vi "DL-Initialize Logging.vi"(0 "Configuration":cluster{"Stop":bool, "Config":T1}, 11 "error in (no error)":errorcluster) -> (3 "RPcoX":refnum<k7>, 4 "task":refnum<k21>, 8 "Npts":i32, 13 "Config.T (s)":dbl, 14 "Config.frame size (s)":dbl, 15 "error out":errorcluster)   [LabVIEW 2020]
uses:
  Typedefs/DL-Configuration.ctl
  Typedefs/DL-Channel Spec.ctl
  <vilib>/DAQmx/create/channels.llb/DAQmx Create Channel (AI-Voltage-Basic).vi
  <vilib>/DAQmx/configure/timing.llb/DAQmx Timing (Sample Clock).vi
  <vilib>/DAQmx/configure/trigger.llb/DAQmx Start Trigger (Digital Edge).vi
  epl-vi-lib/PXI DAQ VIs/TDT VIs/TDT-Signal Bank Action.ctl
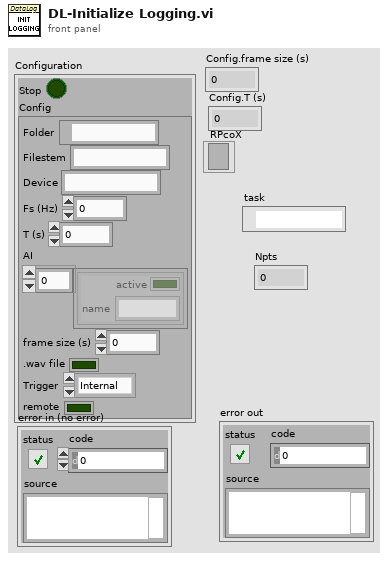
[diagram p1: front panel]
types:
  T1 = typedef "DL-Configuration.ctl" = cluster{"Folder":path, "Filestem":string, "Device":string, "Fs (Hz)":dbl, "T (s)":dbl, "AI":T2[], "frame size (s)":dbl, ".wav file":bool, "Trigger":enum16{"Internal", "External"}, "remote":bool}
  T2 = typedef "DL-Channel Spec.ctl" = cluster{"active":bool, "name":string}
  T3 = typedef "TDT-Signal Bank Action.ctl" = enum16{"Init", "Write", "Read", "Rewrite", "Reset", "Recycle", "Ramp up", "Ramp down", "Zero"}
  T4 = typedef "TDT-Output source.ctl" = cluster{"Device":T5, "Num":i32}
  T5 = typedef "TDT-Device ID.ctl" = enum16{"None", "PA5", "RP2", "RL2", "RA16", "RV8", "RX5", "RX6", "RX7", "RX8", "RZ2", "RZ5", "RZ6"}
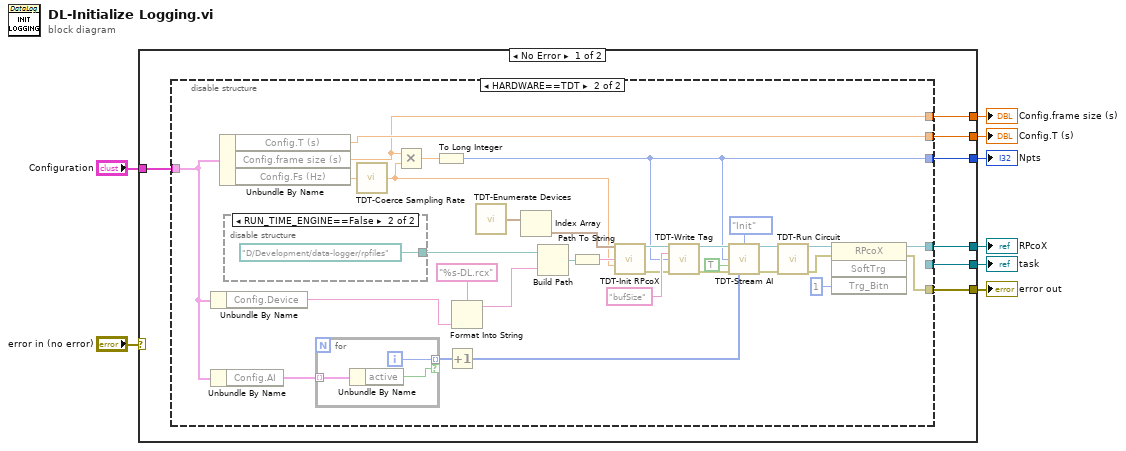
[diagram p0: block diagram]
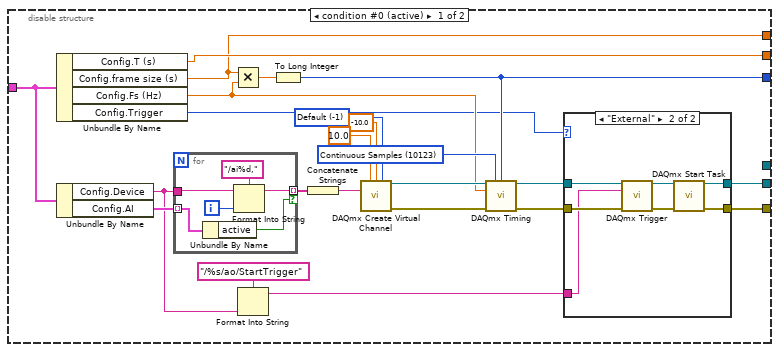
[diagram p2: hidden frame]
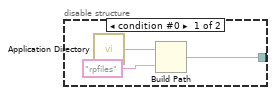
[diagram p4: hidden frame]
diagram:
  n1 = case shown="No Error" "error in (no error)" {
    selector: "error in (no error)" -> [_ w93]
    tunnel: "Configuration" -> [w15 _]
    tunnel: [w13 _] -> w5
    tunnel: [w12 w93] -> w6
    tunnel: [w14 _] -> w4
    tunnel: [w11 _] -> w3
    tunnel: [w10 _] -> w2
    tunnel: [w9 _] -> w1
    frame No Error {
      n2 = disable-structure shown="HARDWARE==TDT" {
        disable-tunnel: w15 -> [w32 w75]
        disable-tunnel: [w29 w54] -> w14
        disable-tunnel: [w27 _] -> w13
        disable-tunnel: [w25 w63] -> w12
        disable-tunnel: [w17 w83] -> w11
        disable-tunnel: [w16 w82] -> w10
        disable-tunnel: [_ w64] -> w9
        frame condition #0 (active) {
          w18 = -1 items=["Default"=-1, "RSE"=10083, "NRSE"=10078, "Differential"=10106, "Pseudodifferential"=12529] ("input terminal configuration")
          w33 = 10123 items=["Finite Samples"=10178, "Continuous Samples"=10123, "Hardware Timed Single Point"=12522] ("sample mode")
          n3 = Unbundle By Name(w32) -> ("Config.T (s)"=w17:dbl, "Config.frame size (s)"=w16:dbl, "Config.Fs (Hz)"=w31:dbl, "Config.Trigger"=w28:enum16{"Internal", "External"})
          n4 = Unbundle By Name(w32) -> ("Config.Device"=w22:string, "Config.AI"=w38:T2[])
          n5 = for {
            tunnel: w38 -> [w49] mode=indexing
            tunnel: w22 -> [w53]
            tunnel: [w50] -> w37 mode=indexing if=w48
            i -> [w51]
            n6 = Unbundle By Name(w49) -> ("active"=w48:bool)
            n7 = Format Into String(format string="/ai%d,", initial string=w53, w51) -> (resulting string=w50:string)  [unwired: 1 in, 1 out]
          }
          n8 = Multiply(x=w16, y=w31) -> (x*y=w30:dbl)
          n9 = Format Into String(format string="/%s/ao/StartTrigger", w22) -> (resulting string=w21:string)  [unwired: 2 in, 1 out]
          n10 = To Long Integer(number=w30) -> (32bit integer=w29:i32)
          n11 = Concatenate Strings(w37) -> (w36:string)
          n12 = call-poly <vilib>:"DAQmx Create Virtual Channel.vi"("maximum value"=10.0, "minimum value"=-10.0, "input terminal configuration"=w18, "physical channels"=w36) -> ("task out"=w35:refnum<k21>, "error out"=w34:errorcluster)  [unwired: 10 in]
          n13 = call-poly <vilib>:"DAQmx Timing.vi"("task/channels in"=w35, "sample mode"=w33, "samples per channel"=w29, "rate"=w31, "error in"=w34) -> ("task out"=w26:refnum<k21>, "error out"=w24:errorcluster)  [unwired: 9 in]
          n14 = case shown="\"External\"" w28 {
            tunnel: [w40 w46] -> w27
            tunnel: w26 -> [w40 w45]
            tunnel: [w39 w47] -> w25
            tunnel: w24 -> [w39 w43]
            tunnel: w21 -> [_ w41]
            frame "Internal", Default {
            }
            frame "External" {
              n15 = call-poly <vilib>:"DAQmx Trigger.vi"("task/channels in"=w45, "source"=w41, "error in"=w43) -> ("task out"=w44:refnum<k21>, "error out"=w42:errorcluster)  [unwired: 11 in]
              n16 = call <vilib>:"DAQmx Start Task.vi"("task/channels in"=w44, "error in"=w42) -> ("task out"=w46:refnum<k21>, "error out"=w47:errorcluster)  [unwired: 12 in]
            }
          }
        }
        frame condition #1 {
          n17 = Unbundle By Name(w75) -> ("Config.Device"=w74:string)
          n18 = Unbundle By Name(w75) -> ("Config.AI"=w85:T2[])
          n19 = Unbundle By Name(w75) -> ("Config.T (s)"=w83:dbl, "Config.frame size (s)"=w82:dbl, "Config.Fs (Hz)"=w81:dbl)
          n20 = disable-structure shown="RUN_TIME_ENGINE==False" {
            disable-tunnel: [w87 path "D:/Development/data-logger/rpfiles"] -> w76
            frame condition #0 {
              n21 = call <vilib>:"Application Directory.vi"() -> ("Application Directory"=w88:path)
              n22 = Build Path(base path=w88, name or relative path="rpfiles") -> (appended path=w87:path)
            }
            frame condition #1 (active) {
            }
          }
          n23 = for {
            tunnel: w85 -> [w92] mode=indexing
            tunnel: [w90] -> w80 mode=indexing if=w91
            i -> [w90]
            n24 = Unbundle By Name(w92) -> ("active"=w91:bool)
          }
          n25 = call "TDT-Coerce Sampling Rate.vi"("Fs (Hz)"=w81) -> ("Coerced"=w67:dbl)
          n26 = Multiply(x=w82, y=w67) -> (x*y=w84:dbl)
          n27 = To Long Integer(number=w84) -> (32bit integer=w54:i32)
          n28 = Increment(x=w80) -> (x+1=w56:i32[])
          n29 = Format Into String(format string="%s-DL.rcx", w74) -> (resulting string=w78:string)  [unwired: 2 in, 1 out]
          n30 = call "TDT-Enumerate Devices.vi"() -> ("Devices"=w70:T4[])  [unwired: 14 in, 1 out]
          n31 = Index Array(array=w70) -> (element=w69:T4)  [unwired: 1 in]
          n32 = Build Path(base path=w76, name or relative path=w78) -> (appended path=w77:path)
          n33 = Path To String(path=w77) -> (string=w68:string)
          n34 = call "TDT-Init RPcoX.vi"("Output"=w69, "RPfilename"=w68, "Sampling rate (Hz)"=w67) -> ("RPcoX"=w73:refnum<k7>, "error out"=w71:errorcluster)  [unwired: 11 in]
          n35 = call "TDT-Write Tag.vi"("RPcox"=w73, "Name"="bufSize", "Value"=w54, "error in"=w71) -> ("RPcox Out"=w61:refnum<k7>, "error out"=w57:errorcluster)  [unwired: 10 in]
          n36 = call "TDT-Stream AI.vi"("RPcox"=w61, "Action"=TDT-Signal_Bank_Action."Init", "Pts Per Read"=w54, "AI only"=TRUE, "error in (no error)"=w57, "AI Channels"=w56) -> ("RPcoX thru"=w59:refnum<k7>, "error out"=w58:errorcluster)  [unwired: 7 in, 1 out]
          n37 = call "TDT-Run Circuit.vi"("RPcoX"=w59, "error in (no error)"=w58) -> ("RPcoX out"=w65:refnum<k7>, "error out"=w62:errorcluster)  [unwired: 12 in]
          n38 = invoke class="RPcoX" method="SoftTrg"(reference=w65, error in=w62, "Trg_Bitn"=1) -> (reference out=w64:refnum<k7>, error out=w63:errorcluster)  [unwired: 1 in, 2 out]
        }
      }
    }
    frame Error {
    }
  }
  "error out" <- w6
  "task" <- w5
  "Npts" <- w4
  "Config.frame size (s)" <- w2
  "Config.T (s)" <- w3
  "RPcoX" <- w1
